vi "testMaxFileSize.vi"(8 "error in (no error)":errorcluster, 11 "TestCase in":refnum<class "Test-File IO.lvclass">=refnum) -> (0 "error out":errorcluster, 3 "TestCase out":refnum<class "Test-File IO.lvclass">)   [LabVIEW 2019, in "Test-File IO.lvclass"]
uses:
  Test-File IO.lvclass
  Log/Event Level.ctl
  TSC Event Logger.lvlib
  Log/Log.lvclass
  Log Sinks/Text File/Text File.lvclass
  9400858f-8242-4f0f-a3a8-0c5d1ac263e7.vi
  C:/Development/Open Source/tsc-event-logger/Log Sinks/Log Sinks.lvclass
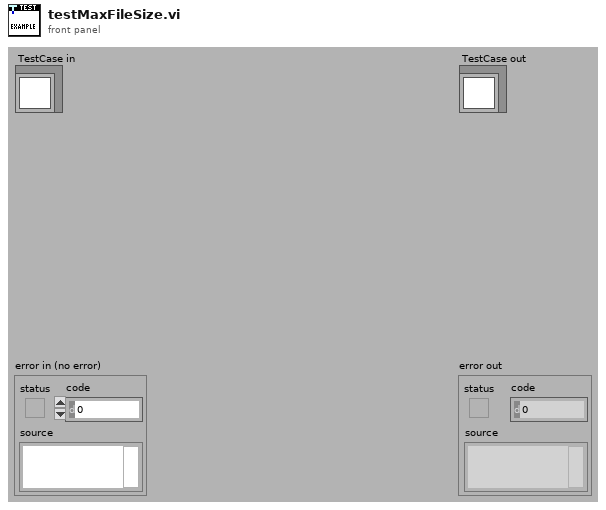
[diagram p1: front panel]
types:
  T1 = typedef "TSC Event Logger.lvlib/Event Level.ctl" = enum16{"OFF", "TRACE", "DEBUG", "INFO", "WARN", "ERROR", "FATAL"}
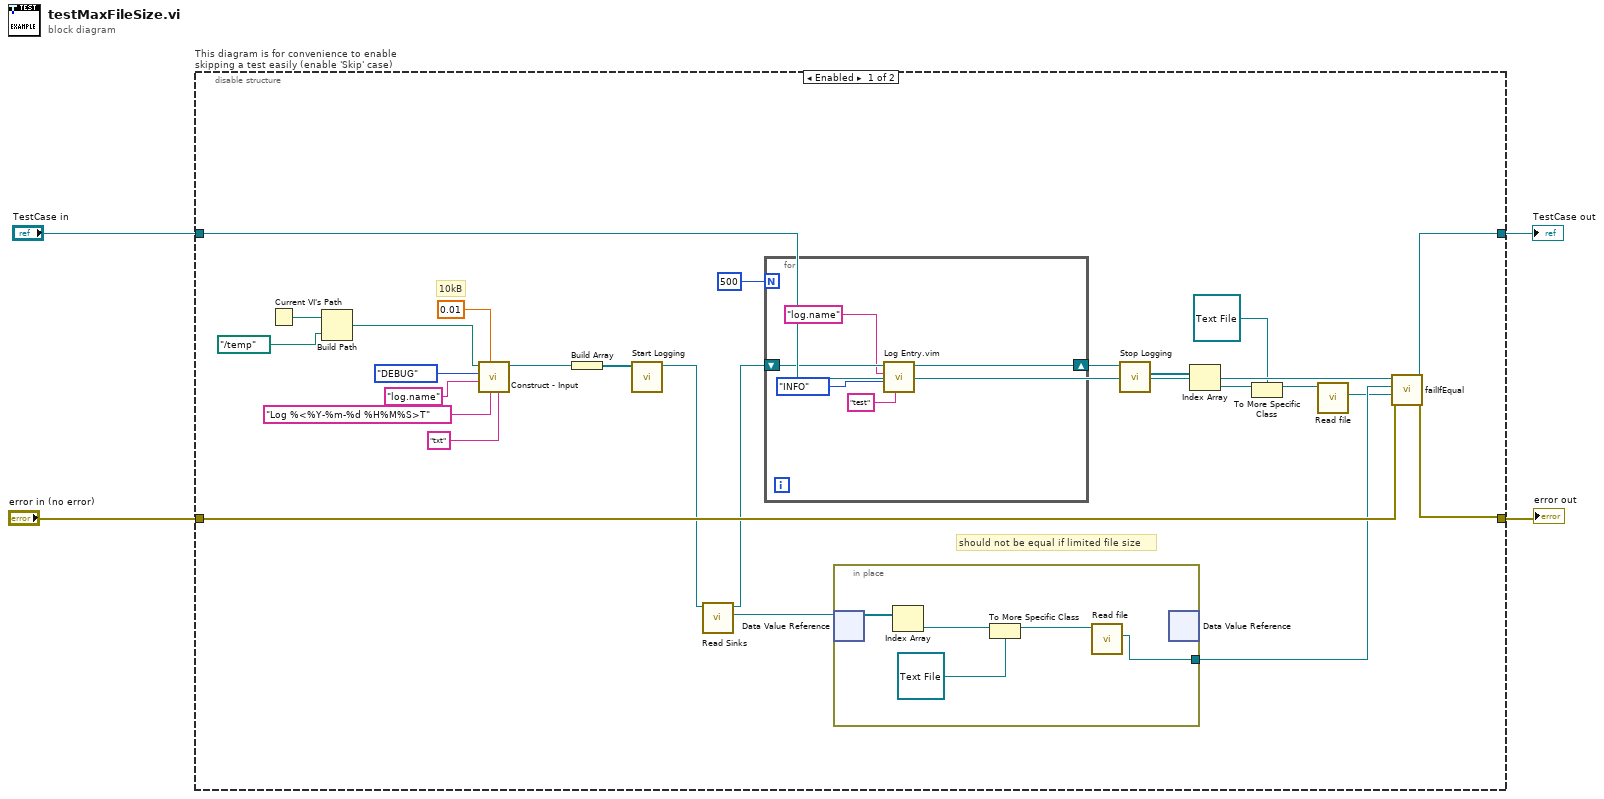
[diagram p0: block diagram]
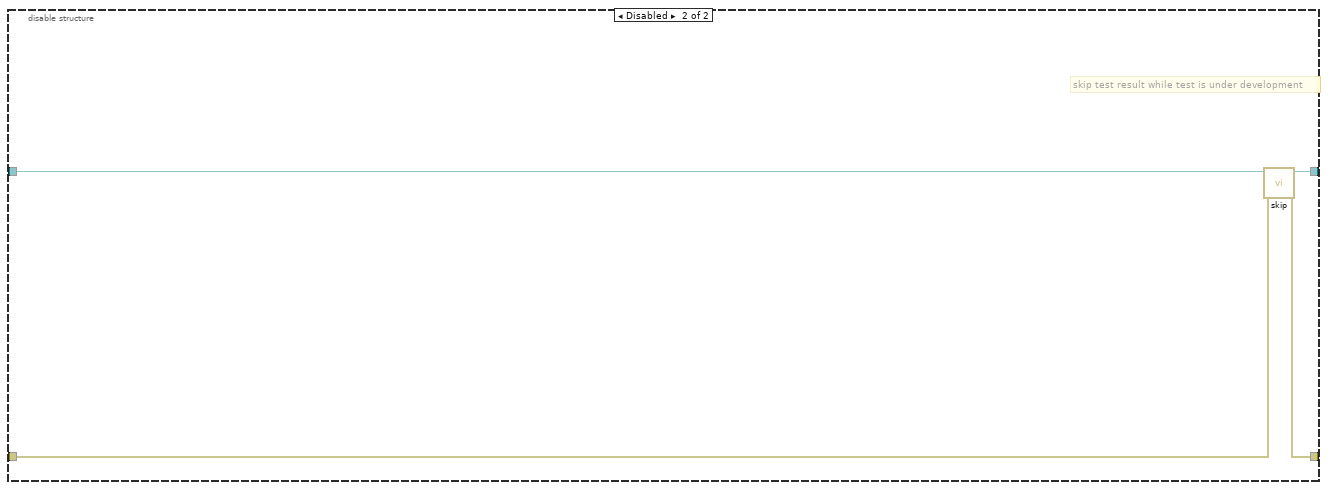
[diagram p2: hidden frame]
diagram:
  n1 = disable-structure "This diagram is for convenience to enable skipping a test easily (enable 'Skip' case)" shown="Enabled" {
    disable-tunnel: "TestCase in" -> [w26 w43]
    disable-tunnel: [w29 w41] -> w1
    disable-tunnel: [w28 w42] -> w3
    disable-tunnel: "error in (no error)" -> [w27 w40]
    frame Enabled {
      # "10kB"
      # "should not be equal if limited file size"
      n2 = Current VI's Path() -> (path=w13:path)
      n3 = Build Path(base path=w13, name or relative path=path "../temp") -> (appended path=w15:path)
      n4 = call "Construct - Input.vi"("extension"="txt", "file name format"="Log %<%Y-%m-%d %H%M%S>T", "Max File Size (MB)"=0.01, "Name"="log.name", "Level"=Event_Level."DEBUG", "log location"=w15) -> ("Text File"=w8:refnum<class "Text File.lvclass">)  [unwired: 4 in, 1 out]
      n5 = Build Array(w8) -> (w7:refnum<class "Text File.lvclass">[])
      n6 = call "Start Logging.vi"("Sinks"=w7) -> ("Logger"=w5:refnum<class "Log.lvclass">)  [unwired: 9 in, 1 out]
      n7 = call "Read Sinks.vi"("Log in"=w5) -> ("Sink DVR Array"=w25:refnum<data-value>, "Log out"=w20:refnum<class "Log.lvclass">)  [unwired: 9 in]
      n8 = for {
        N: 500 -> [_]
        shift-right: [w37] -> w21
        shift-left: w20 -> [w38]
        n9 = call "Log Entry.vim"("Message"="test", "Level"=Event_Level."INFO", "Logger"="log.name", "Log in"=w38) -> ("Log out"=w37:refnum<class "Log.lvclass">)  [unwired: 6 in, 1 out]
      }
      n10 = in-place {
        in-place-border: [w30] -> w24
        n11 = in-place-dvr #1(w25) -> (w34:refnum<class "Log Sinks.lvclass">[])  [unwired: 1 out]
        n12 = Index Array(array=w34) -> (element=w33:refnum<class "Log Sinks.lvclass">)  [unwired: 1 in]
        n13 = To More Specific Class(target class=refnum<class "Text File.lvclass"> refnum ("TSC Event Logger.lvlib:Text File.lvclass"), reference=w33) -> (specific class reference=w32:refnum<class "Text File.lvclass">)  [unwired: 1 in, 1 out]
        n14 = call "Read file.vi"("Text File in"=w32) -> ("file"=w30:refnum<file>)  [unwired: 9 in, 1 out]
        n15 = in-place-dvr #1() -> ()  [unwired: 1 in, 2 out]
      }
      n16 = call "Stop Logging.vi"("Logger"=w21) -> ("sinks"=w16:refnum<class "Log Sinks.lvclass">[])  [unwired: 9 in, 1 out]
      n17 = Index Array(array=w16) -> (element=w19:refnum<class "Log Sinks.lvclass">)  [unwired: 1 in]
      n18 = To More Specific Class(target class=refnum<class "Text File.lvclass"> refnum ("TSC Event Logger.lvlib:Text File.lvclass"), reference=w19) -> (specific class reference=w18:refnum<class "Text File.lvclass">)  [unwired: 1 in, 1 out]
      n19 = call "Read file.vi"("Text File in"=w18) -> ("file"=w22:refnum<file>)  [unwired: 9 in, 1 out]
      n20 = call-dynamic "failIfEqual.vi"("error in (no error)"=w27, "y"=w22, "x"=w24, "TestCase in"=w26) -> ("error out"=w28:errorcluster, "TestCase out"=w29:refnum<class "Test-File IO.lvclass">)  [unwired: 6 in]
    }
    frame Disabled {
      # "skip test result while test is under development"
      n21 = call <vilib>:"skip.vi"("error in (no error)"=w40, "TestCase in"=w43) -> ("error out"=w42:errorcluster, "TestCase out"=w41:refnum<class "Test-File IO.lvclass">)  [unwired: 8 in]
    }
  }
  "error out" <- w3
  "TestCase out" <- w1
